vi "DM Pixel Scan Counter.vi"(2 "Action":T1(ring), 7 "Pixel Scan Parameters In":T2={"Scan Start Pixel"=1, "Scan End Pixel"=1, "Pixel Start Value (-1 to 1)"=-0.5, "Pixel End Value (-1 to 1)"=0.5, "Number of Steps"=0.1}, 11 "Initial Pixel Values (-1 to 1)":dbl[](array[numeric])) -> (4 "Scan Done":bool, 6 "DM Pixel":i32, 10 "Normalized DM Pixel Value":dbl, 15 "Initial Pixel Values OUT":dbl[](array[numeric]))   [LabVIEW 2014]
uses:
  Pixel Scan Parameters.ctl
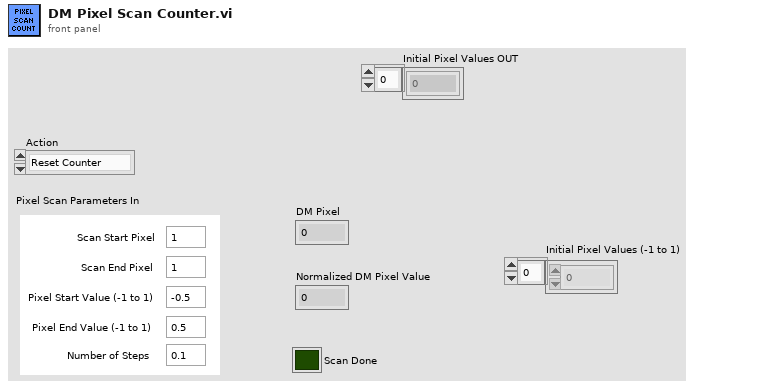
[diagram p1: front panel]
types:
  T1 = enum16{"Reset Counter", "Update Counter", "Get Count"}
  T2 = typedef "Pixel Scan Parameters.ctl" = cluster{"Scan Start Pixel":i32, "Scan End Pixel":i32, "Pixel Start Value (-1 to 1)":dbl, "Pixel End Value (-1 to 1)":dbl, "Number of Steps":dbl}
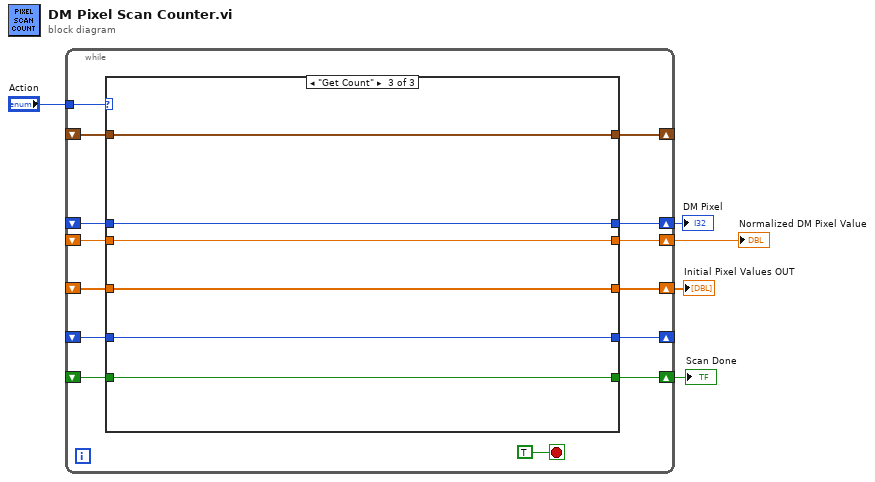
[diagram p0: block diagram]
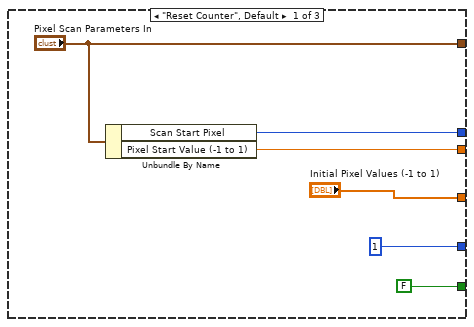
[diagram p2: hidden frame]
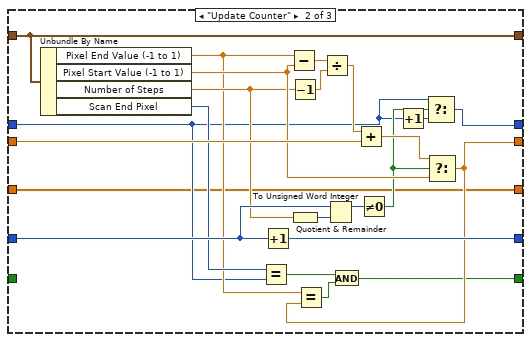
[diagram p3: hidden frame]
diagram:
  n1 = while {
    tunnel: "Action" -> [w18]
    shift-right: [w17] -> _
    shift-left: _ -> [w12]
    shift-right: [w16] -> w4
    shift-left: _ -> [w14]
    shift-right: [w15] -> w3
    shift-left: _ -> [w13]
    shift-right: [w11] -> _
    shift-left: _ -> [w10]
    shift-right: [w9] -> w2
    shift-left: _ -> [w8]
    shift-right: [w7] -> w1
    shift-left: _ -> [w6]
    stop <- TRUE stop-if-true
    n2 = case shown="\"Get Count\"" w18 {
      tunnel: ["Pixel Scan Parameters In" w47 w52] -> w17
      tunnel: [w24 w34 w54] -> w16
      tunnel: [w23 w31 w53] -> w15
      tunnel: w14 -> [_ w27 w54]
      tunnel: w13 -> [_ w45 w53]
      tunnel: w12 -> [_ w47 w52]
      tunnel: [u16 1 w42 w51] -> w11
      tunnel: w10 -> [_ w44 w51]
      tunnel: [FALSE w28 w50] -> w9
      tunnel: w8 -> [_ _ w50]
      tunnel: ["Initial Pixel Values (-1 to 1)" w26 w49] -> w7
      tunnel: w6 -> [_ w26 w49]
      frame "Reset Counter", Default {
        n3 = Unbundle By Name("Pixel Scan Parameters In") -> ("Scan Start Pixel"=w24:i32, "Pixel Start Value (-1 to 1)"=w23:dbl)
      }
      frame "Update Counter" {
        n4 = Unbundle By Name(w47) -> ("Pixel End Value (-1 to 1)"=w32:dbl, "Pixel Start Value (-1 to 1)"=w40:dbl, "Number of Steps"=w38:dbl, "Scan End Pixel"=w33:i32)
        n5 = Equal?(x=w33, y=w27) -> (x = y?=w30:bool)
        n6 = Increment(x=w44) -> (x+1=w42:u16)
        n7 = Subtract(x=w32, y=w40) -> (x-y=w48:dbl)
        n8 = Decrement(x=w38) -> (x-1=w37:dbl)
        n9 = To Unsigned Word Integer(number=w38) -> (unsigned 16bit integer=w43:u16)
        n10 = Divide(x=w48, y=w37) -> (x/y=w46:dbl)
        n11 = Quotient & Remainder(x=w44, y=w43) -> (x-y*floor(x/y)=w41:u16)  [unwired: 1 out]
        n12 = Add(x=w46, y=w45) -> (x+y=w39:dbl)
        n13 = Not Equal To 0?(x=w41) -> (x != 0?=w36:bool)
        n14 = Increment(x=w27) -> (x+1=w35:i32)
        n15 = Select(t=w27, s=w36, f=w35) -> (s? t:f=w34:i32)
        n16 = Select(t=w39, s=w36, f=w40) -> (s? t:f=w31:dbl)
        n17 = Equal?(x=w32, y=w31) -> (x = y?=w29:bool)
        n18 = And(x=w30, y=w29) -> (x .and. y?=w28:bool)
      }
      frame "Get Count" {
      }
    }
  }
  "DM Pixel" <- w4
  "Normalized DM Pixel Value" <- w3
  "Scan Done" <- w2
  "Initial Pixel Values OUT" <- w1
